vi "calculateGraphData.vi"(7 "Online Buffer (1000)":i32=1000, 8 "error in":errorcluster, 9 "Offset in":i64, 10 "DataBuffers in":dbl[][](array[numeric]), 11 "GraphData in":cluster{dbl[], dbl[]}[](array[cluster])) -> (0 "error out":errorcluster, 3 "GraphData out":cluster{dbl[], dbl[]}[](array[cluster]))   [LabVIEW 2022 SP3, in "MultiReader.lvlib"]
uses:
  <instrlib>/openDAQ/Examples/MultiReader/MultiReader.lvlib
  <instrlib>/openDAQ/Public/Classes/daqUtils/daqUtils.lvlib
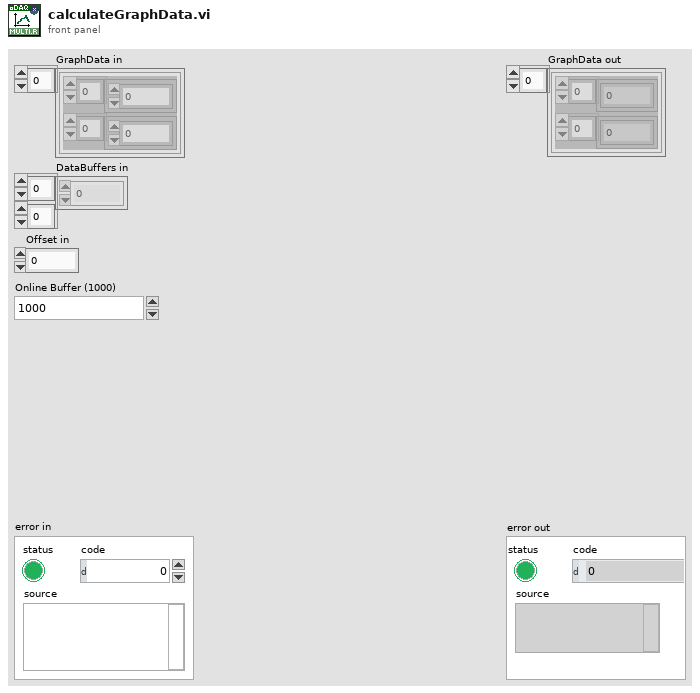
[diagram p1: front panel]
types:
  T1 = enum16{"init", "read", "set sampleRate", "set ruleStart", "set ruleDelta", "set referenceDomainOffset", "set origin", "set unitSymbol", "set resNum", "set resDen", " calculate sampleRate"}
  T2 = typedef "openDAQ.lvlib/DomainMetadata.ctl" = cluster{"sampleRate":i64, "ruleStart":i64, "ruleDelta":i64, "referenceDomainOffset":i64, "origin":timestamp, "unitSymbol":string, "resNum":i64, "resDen":i64}
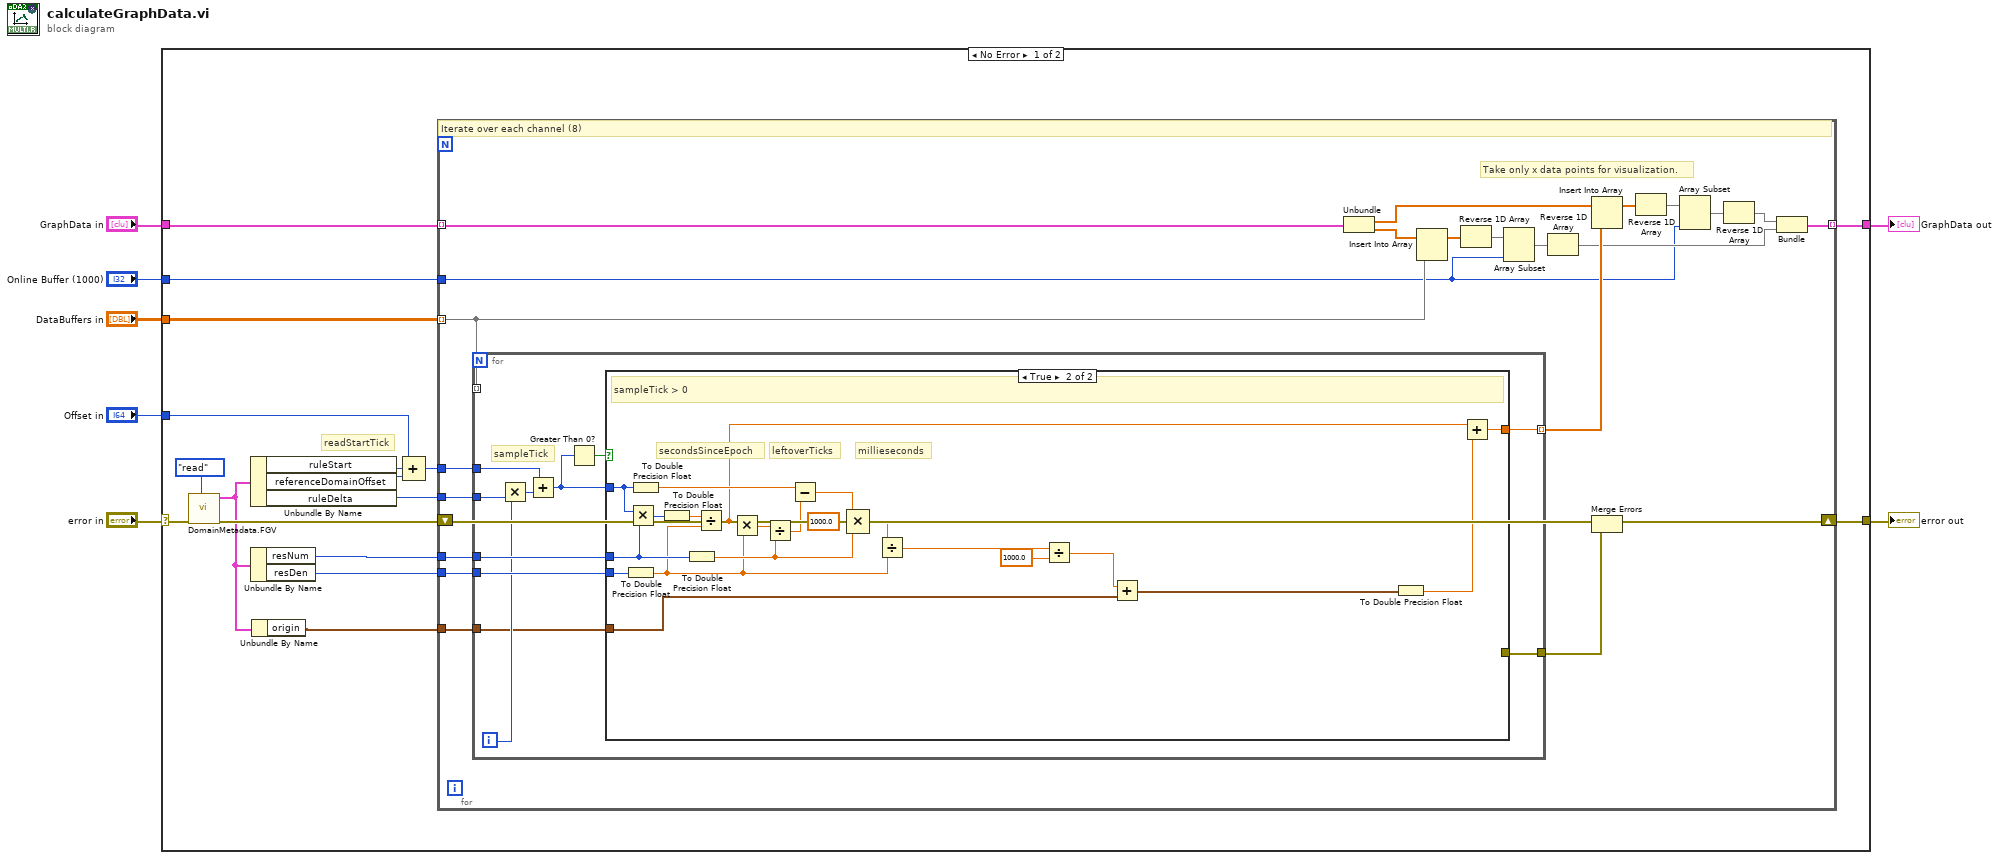
[diagram p0: block diagram]
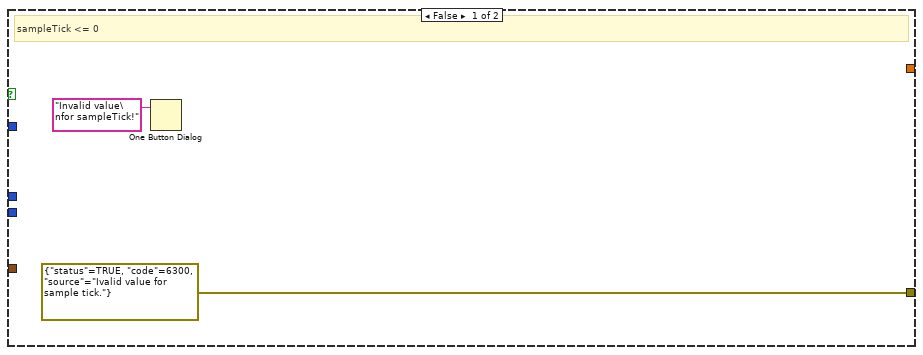
[diagram p2: hidden frame]
diagram:
  n1 = case shown="No Error" "error in" {
    selector: "error in" -> [w10 w83]
    tunnel: [w20 w83] -> w7
    tunnel: "DataBuffers in" -> [w14 _]
    tunnel: "Offset in" -> [w13 _]
    tunnel: "GraphData in" -> [w12 w82]
    tunnel: [w11 w82] -> w3
    tunnel: "Online Buffer (1000)" -> [w9 _]
    frame No Error {
      # "readStartTick"
      n2 = call <instrlib>:"DomainMetadata.FGV.vi"("Case Select"=T1."read", "error in"=w10) -> ("error out"=w21:errorcluster, "DomainMetadata out"=w15:T2)  [unwired: 8 in]
      n3 = Unbundle By Name(w15) -> ("ruleStart"=w23:i64, "referenceDomainOffset"=w22:i64, "ruleDelta"=w18:i64)
      n4 = Unbundle By Name(w15) -> ("resNum"=w17:i64, "resDen"=w16:i64)
      n5 = Unbundle By Name(w15) -> ("origin"=w8:timestamp)
      n6 = Compound Arithmetic op=ADD(w13, w23, w22) -> (w19:i64)
      n7 = for {
        shift-right: [w41] -> w20
        shift-left: w21 -> [w43]
        tunnel: w19 -> [w46]
        tunnel: w18 -> [w47]
        tunnel: w17 -> [w45]
        tunnel: w16 -> [w44]
        tunnel: w14 -> [w27] mode=indexing
        tunnel: [w39] -> w11 mode=indexing
        tunnel: w12 -> [w38] mode=indexing
        tunnel: w9 -> [w26]
        tunnel: w8 -> [w25]
        # "Take only x data points for visualization."
        # "Iterate over each channel (8)"
        n8 = for {
          tunnel: w47 -> [w58]
          tunnel: w46 -> [w56]
          tunnel: w45 -> [w54]
          tunnel: w44 -> [w53]
          tunnel: [w51] -> w42
          tunnel: w27 -> [_] mode=indexing
          tunnel: [w49] -> w40 mode=indexing
          tunnel: w25 -> [w48]
          i -> [w50]
          # "sampleTick"
          n9 = Multiply(x=w50, y=w58) -> (x*y=w57:i64)
          n10 = Add(x=w56, y=w57) -> (x+y=w52:i64)
          n11 = Greater Than 0?(x=w52) -> (x > 0?=w55:bool)
          n12 = case shown="True" w55 {
            tunnel: w54 -> [_ w77]
            tunnel: w53 -> [_ w79]
            tunnel: w52 -> [_ w76]
            tunnel: [errorcluster {"status"=TRUE, "code"=6300, "source"="Ivalid value for sample tick."} ("error in (no error)") _] -> w51
            tunnel: [_ w65] -> w49
            tunnel: w48 -> [_ w62]
            frame False {
              # "sampleTick <= 0"
              n13 = One Button Dialog(message="Invalid value\nfor sampleTick!") -> ()  [unwired: 1 in, 1 out]
            }
            frame True {
              # "millieseconds"
              # "leftoverTicks"
              # "secondsSinceEpoch"
              # "sampleTick > 0"
              n14 = To Double Precision Float(number=w79) -> (double precision float=w69:dbl)
              n15 = Multiply(x=w76, y=w77) -> (x*y=w81:i64)
              n16 = To Double Precision Float(number=w76) -> (double precision float=w74:dbl)
              n17 = To Double Precision Float(number=w81) -> (double precision float=w80:dbl)
              n18 = To Double Precision Float(number=w77) -> (double precision float=w71:dbl)
              n19 = Divide(x=w80, y=w69) -> (x/y=w67:dbl)
              n20 = Multiply(x=w67, y=w69) -> (x*y=w78:dbl)
              n21 = Divide(x=w78, y=w71) -> (x/y=w75:dbl)
              n22 = Subtract(x=w74, y=w75) -> (x-y=w73:dbl)
              n23 = Compound Arithmetic op=MULTIPLY(w73, 1000.0 ("x/y"), w71) -> (w70:dbl)
              n24 = Divide(x=w70, y=w69) -> (x/y=w68:dbl)
              n25 = Divide(x=w68, y=1000.0) -> (x/y=w63:dbl)
              n26 = Add(x=w63, y=w62) -> (x+y=w61:timestamp)
              n27 = To Double Precision Float(number=w61) -> (double precision float=w66:dbl)
              n28 = Add(x=w67, y=w66) -> (x+y=w65:dbl)
            }
          }
        }
        n29 = Unbundle(w38) -> (w37:dbl[], w36:dbl[])
        n30 = Insert Into Array(array=w36, new element=w27) -> (w35:dbl[])  [unwired: 1 in]
        n31 = Reverse 1D Array(array=w35) -> (reversed array=w31:dbl[])
        n32 = Array Subset(array=w31, length=w26) -> (w34:dbl[])  [unwired: 1 in]
        n33 = Reverse 1D Array(array=w34) -> (reversed array=w30:dbl[])
        n34 = Insert Into Array(array=w37, new element=w40) -> (w33:dbl[])  [unwired: 1 in]
        n35 = Merge Errors(w43, w42) -> (w41:errorcluster)
        n36 = Reverse 1D Array(array=w33) -> (reversed array=w29:dbl[])
        n37 = Array Subset(array=w29, length=w26) -> (w32:dbl[])  [unwired: 1 in]
        n38 = Reverse 1D Array(array=w32) -> (reversed array=w28:dbl[])
        n39 = Bundle(w28, w30) -> (w39:cluster{dbl[], dbl[]})  [unwired: 1 in]
      }
    }
    frame Error {
    }
  }
  "error out" <- w7
  "GraphData out" <- w3
